vi "get_runningAgents.vi"(0 "Host_Reference":refnum<class "HGF_Reference.lvclass">, 2 "timeout in ms (-1)":i32=-1, 5 "error in (no error)":errorcluster) -> (14 "dup Host_Reference":refnum<class "HGF_Reference.lvclass">, 16 "Running Agents":string[](array[string]), 19 "error out":errorcluster)   [LabVIEW 2009, in "MoAgSy.lvlib" / "MoAgSy_Host.lvclass"]
doc: "<B>public</B> VI returns a list of the referenced Hosts running agents.\n\nF.Berck@gsi.de\nGSI Darmstadt 2009"
uses:
  MoAgSy_Host.lvclass
  HGF_BaseClasses/HGF_Reference/HGF_Reference.lvclass
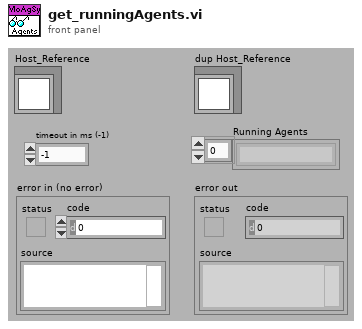
[diagram p1: front panel]
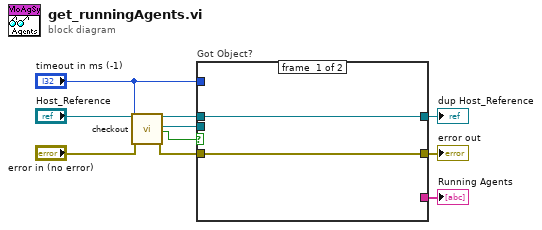
[diagram p0: block diagram]
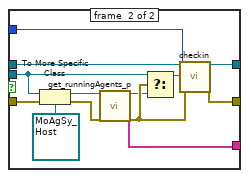
[diagram p2: hidden frame]
diagram:
  n1 = call "checkout.vi"("HGF_Reference"="Host_Reference", "timeout in ms (-1)"="timeout in ms (-1)", "error in (no error)"="error in (no error)") -> ("dup HGF_Reference"=w5:refnum<class "HGF_Reference.lvclass">, "Object"=w4:refnum<class>, "got object?"=w2:bool, "error out"=w3:errorcluster)  [unwired: 13 out]
  n2 = case "Got Object?" shown="True" w2 {
    tunnel: w4 -> [_ w19]
    tunnel: w5 -> [w12 w24]
    tunnel: [w12 w23] -> w9
    tunnel: "timeout in ms (-1)" -> [_ w22]
    tunnel: [w11 w21] -> w8
    tunnel: w3 -> [w11 w20]
    tunnel: [_ w13] -> w1
    frame #0 {
    }
    frame #1 {
      n3 = To More Specific Class(target class=refnum<class "MoAgSy_Host.lvclass"> refnum ("MoAgSy.lvlib:MoAgSy_Host.lvclass"), reference=w19, error in=w20) -> (specific class reference=w15:refnum<class "MoAgSy_Host.lvclass">, error out=w17:errorcluster)
      n4 = call "get_runningAgents_p.vi"("MoAgSy_Host"=w15, "error in (no error)"=w17) -> ("dup MoAgSy_Host"=w14:refnum<class "MoAgSy_Host.lvclass">, "Running Agents"=w13:string[], "error out"=w16:errorcluster)  [unwired: 15 out]
      n5 = Select(t=w19, s=w16, f=w14) -> (s? t:f=w18:refnum<class>)
      n6 = call "checkin.vi"("HGF_Reference"=w24, "Object"=w18, "timeout /ms (-1)"=w22, "error in (no error)"=w16) -> ("dup HGF_Reference"=w23:refnum<class "HGF_Reference.lvclass">, "error out"=w21:errorcluster)  [unwired: 14 out]
    }
  }
  "dup Host_Reference" <- w9
  "error out" <- w8
  "Running Agents" <- w1
